vi "checkMotorOverheat.vi"(8 "error in (no error)":errorcluster, 11 "Model in":refnum<class "Model.lvclass">) -> (0 "error out":errorcluster, 3 "Model out":refnum<class "Model.lvclass">)   [LabVIEW 2013, in "Model.lvclass"]
uses:
  Model.lvclass
  Model.lvclass/Model.ctl
  ApplicationElements/TemperatureSensor/MotorTemperatureSensor/MotorTemperatureSensor.lvclass
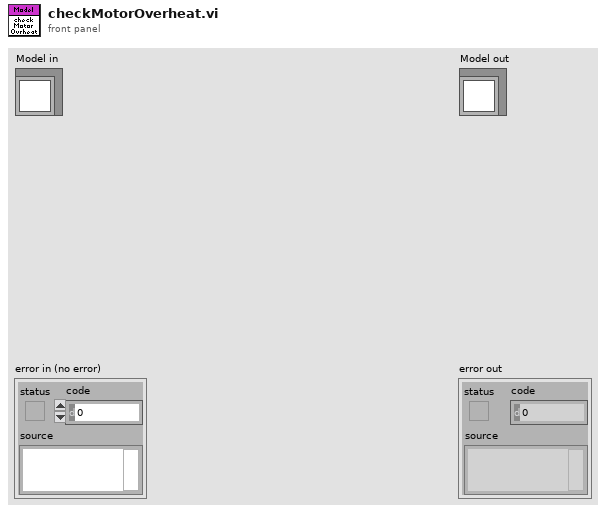
[diagram p1: front panel]
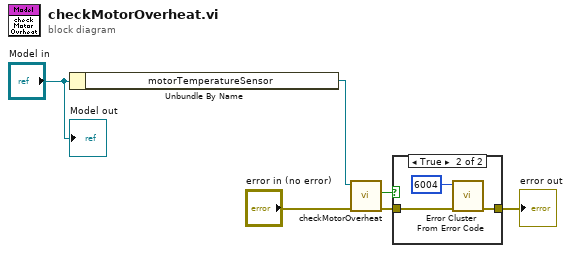
[diagram p0: block diagram]
diagram:
  n1 = Unbundle By Name("Model in") -> ("motorTemperatureSensor"=w5:refnum<class "MotorTemperatureSensor.lvclass">)
  n2 = call "checkMotorOverheat.vi"("error in (no error)"="error in (no error)", "MotorTemperatureSensor in"=w5) -> ("error out"=w1:errorcluster, "motorOverheatActiveIsTrue"=w3:bool)  [unwired: 7 in, 1 out]
  n3 = case shown="True" w3 {
    tunnel: w1 -> [w7 w10]
    tunnel: [w7 w9] -> w6
    frame False {
    }
    frame True {
      n4 = call <vilib>:"Error Cluster From Error Code.vi"("error in (no error)"=w10, "error code (0)"=6004) -> ("error out"=w9:errorcluster)  [unwired: 7 in]
    }
  }
  "error out" <- w6
  "Model out" <- "Model in"
